vi "Initialize.vi"(8 "error in (no error)":errorcluster, 10 "Application":enum16{"TC", "FP"}(ring), 11 "FP-TC-Shared in":refnum<class "FP-TC-Shared.lvclass">) -> (0 "error out":errorcluster, 3 "FP-TC-Shared out":refnum<class "FP-TC-Shared.lvclass">)   [LabVIEW 2019, in "FP-TC-Shared.lvclass"]
uses:
  FP-TC-Shared.lvclass
  FP-TC-Shared.lvclass/FP-TC-Shared.ctl
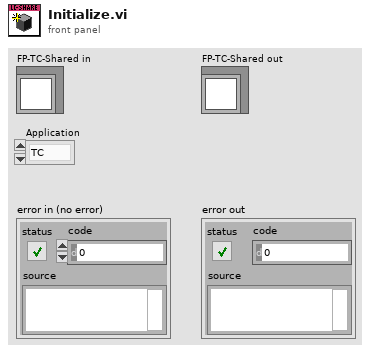
[diagram p1: front panel]
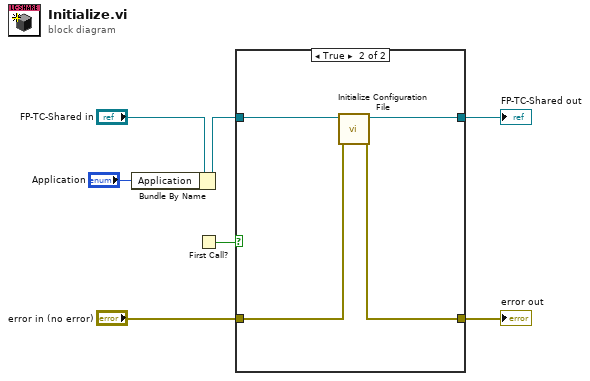
[diagram p0: block diagram]
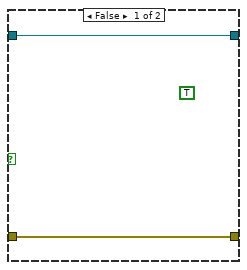
[diagram p2: hidden frame]
diagram:
  n1 = Bundle By Name(cluster="FP-TC-Shared in", "Application"="Application") -> (w2:refnum<class "FP-TC-Shared.lvclass">)
  n2 = First Call?() -> (First Call?: T/F=w7:bool)
  n3 = case shown="True" w7 {
    tunnel: [w9 w11] -> w4
    tunnel: [w8 w12] -> w5
    tunnel: w2 -> [w8 w13]
    tunnel: "error in (no error)" -> [w9 w10]
    frame False {
      (unwired) TRUE ("Last State Known")
    }
    frame True {
      n4 = call "Initialize Configuration File.vi"("error in (no error)"=w10, "FP-TC-Shared in"=w13) -> ("error out"=w11:errorcluster, "FP-TC-Shared out"=w12:refnum<class "FP-TC-Shared.lvclass">)  [unwired: 8 in]
    }
  }
  "FP-TC-Shared out" <- w5
  "error out" <- w4
